vi "Login.vi"(8 "error in (no error)":errorcluster, 11 "reference in":refnum<class "Test_Template.lvclass">) -> (0 "error out":errorcluster, 1 "ok":bool, 3 "reference in":refnum<class "Test_Template.lvclass">)   [LabVIEW 2017]
uses:
  Test_Template.lvclass
  Components/MES_Base.lvlibp/MES_Base.lvclass
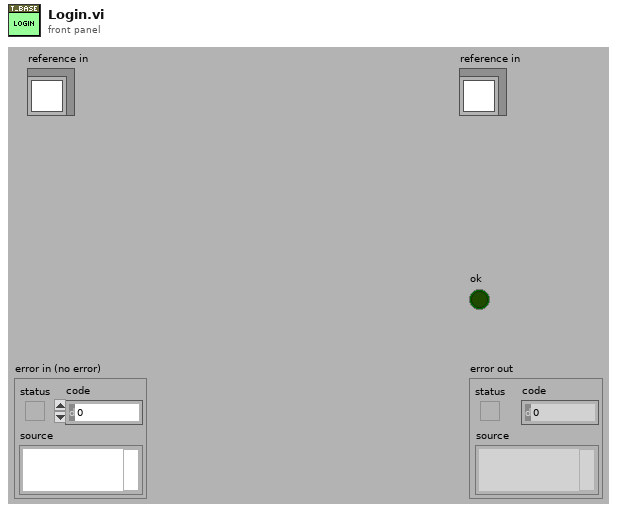
[diagram p1: front panel]
types:
  T1 = typedef "Test_Template.lvlib/Test_Template.lvclass/ObjectAttributes.ctl" = cluster{"Config":T2}
  T2 = typedef "Test_Template.lvlib/Test_Template.lvclass/Config.ctl" = cluster{"default":string}
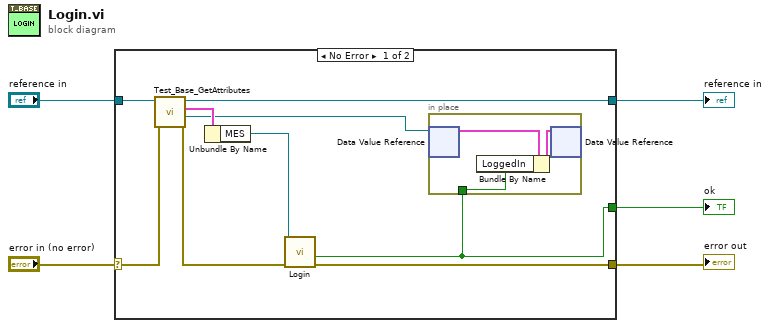
[diagram p0: block diagram]
diagram:
  n1 = case shown="No Error" "error in (no error)" {
    selector: "error in (no error)" -> [w14 w19]
    tunnel: [w8 w19] -> w4
    tunnel: [w11 w18] -> w2
    tunnel: "reference in" -> [w12 w18]
    tunnel: [w6 _] -> w1
    frame No Error {
      n2 = call "Test_Base_GetAttributes.vi"("error in (no error)"=w14, "reference in"=w12) -> ("error out"=w9:errorcluster, "DataRef"=w7:refnum<data-value>, "Data"=w13:T1, "reference out"=w11:refnum<class "Test_Template.lvclass">)  [unwired: 6 in]
      n3 = Unbundle By Name(w13) -> ("MES"=w10:refnum<class "MES_Base.lvclass">)
      n4 = call-dynamic "Login.vi"("error in (no error)"=w9, "reference in"=w10) -> ("error out"=w8:errorcluster, "OK"=w6:bool)  [unwired: 6 in, 1 out]
      n5 = in-place {
        in-place-border: w6 -> [w15]
        n6 = in-place-dvr #1(w7) -> (w17:T1)  [unwired: 1 out]
        n7 = Bundle By Name(cluster=w17, "LoggedIn"=w15) -> (w16:T1)
        n8 = in-place-dvr #1(w16) -> ()  [unwired: 2 out]
      }
    }
    frame Error {
    }
  }
  "error out" <- w4
  "reference in" <- w2
  "ok" <- w1
